vi "Query Current Calibration Factors (RAM).vi"(0 "VISA resource name":refnum<visa-resource-name>, 11 "error in (no error)":errorcluster) -> (4 "VISA resource name out":refnum<visa-resource-name>, 6 "Current Calibration Factors":T1, 15 "error out":errorcluster)   [LabVIEW 2012, in "NH Research Regenerative Test Series.lvlib"]
doc: "This command returns the current calibration factors in RAM."
uses:
  <instrlib>/NH Research Regenerative Test Series/NH Research Regenerative Test Series.lvlib
  <instrlib>/NH Research Regenerative Test Series/Public/Utility/Calibration/Calibration Factors.ctl
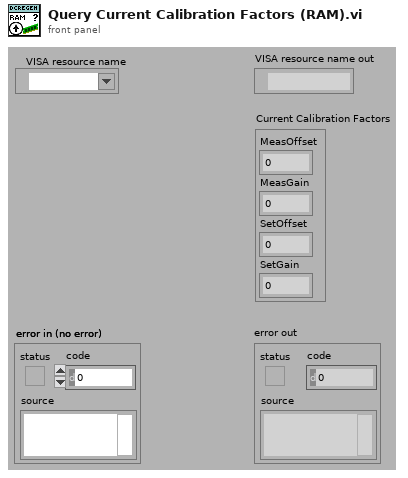
[diagram p1: front panel]
types:
  T1 = typedef "NH Research Regenerative Test Series.lvlib/Calibration Factors.ctl" = cluster{"MeasOffset":dbl, "MeasGain":dbl, "SetOffset":dbl, "SetGain":dbl}
  T2 = cluster{"[0]":dbl, "[1]":dbl, "[2]":dbl, "[3]":dbl}
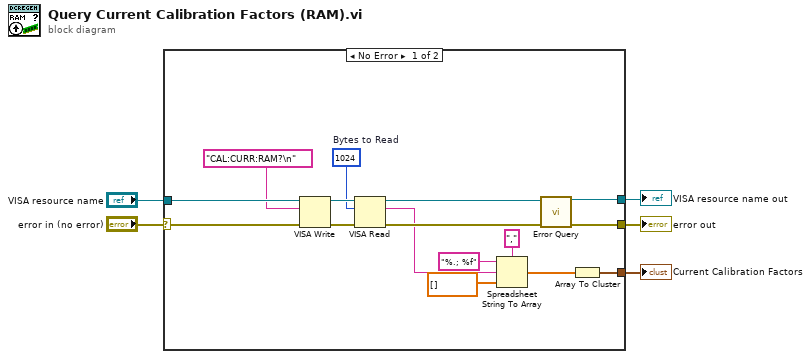
[diagram p0: block diagram]
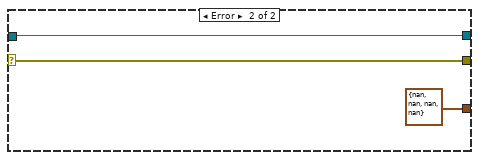
[diagram p2: hidden frame]
diagram:
  n1 = case shown="No Error" "error in (no error)" {
    selector: "error in (no error)" -> [w7 w24]
    tunnel: [w19 w24] -> w4
    tunnel: [w21 w23] -> w2
    tunnel: "VISA resource name" -> [w20 w23]
    tunnel: [w8 T1 {"MeasOffset"=nan, "MeasGain"=nan, "SetOffset"=nan, "SetGain"=nan} ("Calibration Factors")] -> w1
    frame No Error {
      w15 = u32 1024  # Bytes to Read
      n2 = VISA Write(VISA resource name=w20, write buffer="CAL:CURR:RAM?\n", error in (no error)=w7) -> (VISA resource name out=w16:refnum<visa-resource-name>, error out=w17:errorcluster)  [unwired: 1 out]
      n3 = VISA Read(VISA resource name=w16, byte count=w15, error in (no error)=w17) -> (VISA resource name out=w18:refnum<visa-resource-name>, read buffer=w10:string, error out=w11:errorcluster)  [unwired: 1 out]
      n4 = Spreadsheet String To Array(delimiter (Tab)=",", format string="%.; %f", spreadsheet string=w10, array type (2D Dbl)=dbl[] []) -> (array=w9:dbl[])
      n5 = call <instrlib>:"Error Query.vi"("VISA resource name"=w18, "error in (no error)"=w11) -> ("VISA resource name out"=w21:refnum<visa-resource-name>, "error out"=w19:errorcluster)  [unwired: 10 in, 2 out]
      n6 = Array To Cluster(array=w9) -> (cluster=w8:T2)
    }
    frame Error {
    }
  }
  "error out" <- w4
  "VISA resource name out" <- w2
  "Current Calibration Factors" <- w1
